vi "LNLS Control FOFB Configuration In.vi"() -> ()   [LabVIEW 2011, in "Controller Global Variables.lvlib"]
uses:
  Controller Global Variables.lvlib
  Types Definitions/Type Control FOFB Configuration In.ctl
  Types Definitions/Type Operation Mode State.ctl
  Type Definitions.lvlib
panel:
  in  "LNLS Control FOFB Configuration In":T1={"Status"=0, "Operation Mode"=enum."Manual Mode", "Horizontal Gain"=0.0, "Vertical Gain"=0.0, "Selected Reference Orbit"=0, "Selected Correction Matrix"=0, "Selected FPGA Filters"=0, "Horizontal Distortion Threshold"=0.0, "Vertical Distortion Threshold"=0.0, "Fast Command Enabled"=FALSE, "Update Reference Orbit"=FALSE, "Update Contoller Configuration"=FALSE}
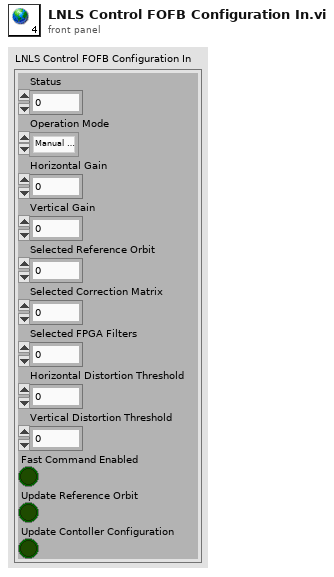
[diagram p1: front panel]
types:
  T1 = typedef "Type Definitions.lvlib/Type Control FOFB Configuration In.ctl" = cluster{"Status":u16, "Operation Mode":T2, "Horizontal Gain":sgl, "Vertical Gain":sgl, "Selected Reference Orbit":i32, "Selected Correction Matrix":i32, "Selected FPGA Filters":i32, "Horizontal Distortion Threshold":sgl, "Vertical Distortion Threshold":sgl, "Fast Command Enabled":bool, "Update Reference Orbit":bool, "Update Contoller Configuration":bool}
  T2 = typedef "Type Definitions.lvlib/Type Operation Mode State.ctl" = enum8{"Idle Mode", "Manual Mode", "FOFB Mode"}
diagram:
